vi "Raycaster_RunDDA.vi"(10 "Map Address":u32, 11 "DDA Calculation In":T1) -> (3 "DDA Calculation Out":T1)   [LabVIEW 2020]
uses:
  Controls/Raycaster_DDACalcs.ctl
  Controls/Raycaster_WallColumnAxis.ctl
  Globals/FGV_TileVisibleEnum.ctl
  Map_GetMaps.vi
  <vilib>/Utility/file.llb/Application Directory.vi
  <vilib>/rvi/DataTransferAndStorage/Container/XNode/niFpgaContainer.xnode
  <vilib>/rvi/Memory/Memory_Emulation/nirvimemoryFastEmulation.vi
  <vilib>/rvi/Memory/Memory_Emulation/nirvimemoryEmulation.vi
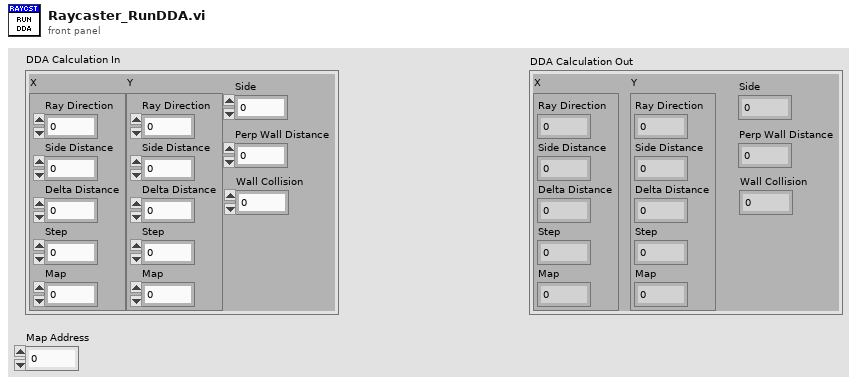
[diagram p1: front panel]
types:
  T1 = typedef "Raycaster_DDACalcs.ctl" = cluster{"X":T2, "Y":T2, "Side":u8, "Perp Wall Distance":fxp<+/-,32,16>, "Wall Collision":u8}
  T2 = typedef "Raycaster_WallColumnAxis.ctl" = cluster{"Ray Direction":fxp<+/-,32,16>, "Side Distance":fxp<+/-,32,16>, "Delta Distance":fxp<+/-,32,16>, "Step":i16, "Map":i16}
  T3 = typedef "FGV_TileVisibleEnum.ctl" = enum16{"Reset", "Set Value", "Read Value"}
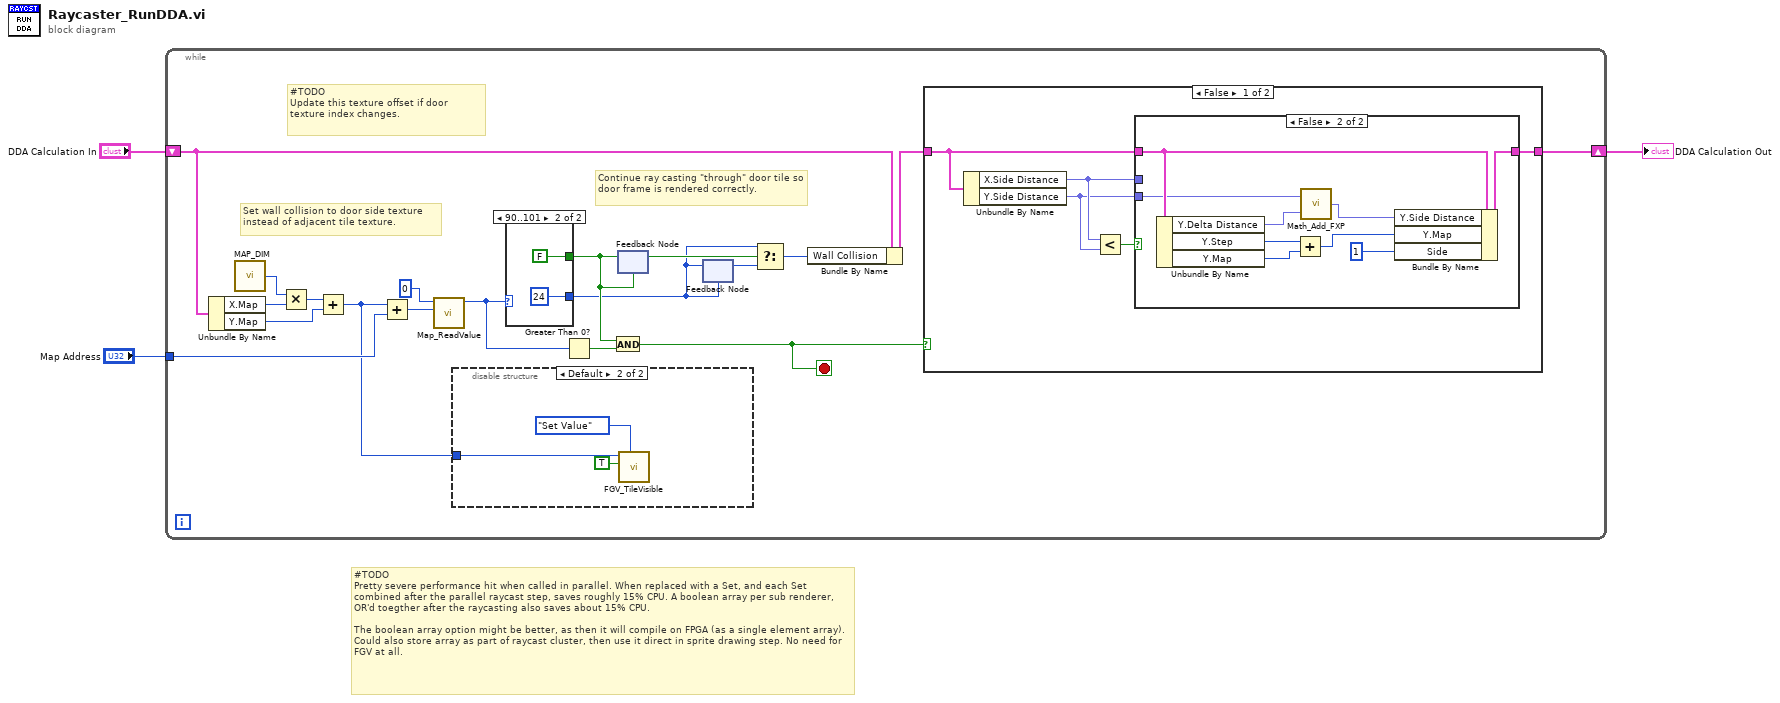
[diagram p0: block diagram]
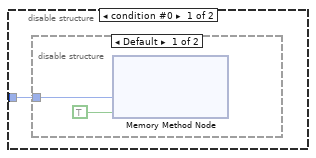
[diagram p2: hidden frame]
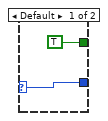
[diagram p4: hidden frame]
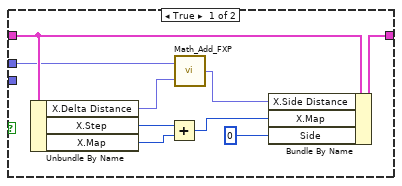
[diagram p5: hidden frame]
diagram:
  # "#TODO\nPretty severe performance hit when called in parallel. When replaced with a Set, and each Set combined after the parallel raycast step, saves roughly 15% CPU. A boolean array per sub renderer, OR'd toegther after the raycasting also saves about 15% CPU.\n\nThe boolean array option might be better, as then it will compile on FPGA (as a single element array). Could also store array as part of raycast cluster, then use it direct in sprite drawing step. No need for FGV at all."
  n1 = while {
    shift-right: [w15] -> w2
    shift-left: "DDA Calculation In" -> [w11]
    tunnel: "Map Address" -> [w6]
    stop <- w9 stop-if-true
    # "#TODO\nUpdate this texture offset if door texture index changes."
    # "Set wall collision to door side texture instead of adjacent tile texture."
    # "Continue ray casting \"through\" door tile so door frame is rendered correctly."
    n2 = Unbundle By Name(w11) -> ("X.Map"=w22:i16, "Y.Map"=w20:i16)
    n3 = call "MAP_DIM.vi"() -> ("MAP_DIM"=w19:i16)
    n4 = Multiply(x=w19, y=w22) -> (x*y=w21:i16)
    n5 = Add(x=w21, y=w20) -> (x+y=w4:i16)
    n6 = Add(x=w4, y=w6) -> (x+y=w5:u32)
    n7 = call "Map_ReadValue.vi"("Address"=w5, "Plane"=u8 0) -> ("Value"=w16:u8)  [unwired: 9 in]
    n8 = disable-structure shown="Default" {
      disable-tunnel: w4 -> [w23 w27]
      frame condition #0 {
        n9 = disable-structure shown="Default" {
          disable-tunnel: w23 -> [w25 _]
          frame condition #0 (active) {
            n10 = xnode ("Memory Method Node")("Address"=w25, "Data"=TRUE) -> ()  [unwired: 1 in, 1 out]
          }
          frame condition #1 {
          }
        }
      }
      frame condition #1 (active) {
        n11 = call "FGV_TileVisible.vi"("Tile Visible FGV"=FGV_TileVisibleEnum."Set Value", "Value"=TRUE, "Index"=w27) -> ()  [unwired: 8 in, 1 out]
      }
    }
    n12 = case shown="90..101" w16 {
      selector: w16 -> [w30 _]
      tunnel: [w30 u8 24 ("Value")] -> w7
      tunnel: [TRUE FALSE] -> w8
      frame Default {
      }
      frame 90..101 {
      }
    }
    n13 = Greater Than 0?(x=w16) -> (x > 0?=w17:bool)
    n14 = And(x=w8, y=w17) -> (x .and. y?=w9:bool)
    n15 = feedback #1(w8) -> (w13:bool)
    n16 = feedback-in #1(w8) -> ()
    n17 = feedback #2(w7) -> (w14:u8)
    n18 = feedback-in #2(w7) -> ()
    n19 = Select(t=w7, s=w13, f=w14) -> (s? t:f=w12:u8)
    n20 = Bundle By Name(cluster=w11, "Wall Collision"=w12) -> (w10:T1)
    n21 = case shown="False" w9 {
      tunnel: w10 -> [w34 w56]
      tunnel: [w33 w56] -> w15
      frame False {
        n22 = Unbundle By Name(w34) -> ("X.Side Distance"=w36:fxp<+/-,32,16>, "Y.Side Distance"=w35:fxp<+/-,32,16>)
        n23 = Less?(x=w36, y=w35) -> (x < y?=w37:bool)
        n24 = case shown="False" w37 {
          tunnel: w34 -> [w46 w55]
          tunnel: w36 -> [w40 _]
          tunnel: [w41 w50] -> w33
          tunnel: w35 -> [_ w49]
          frame True {
            n25 = Unbundle By Name(w46) -> ("X.Delta Distance"=w39:fxp<+/-,32,16>, "X.Step"=w45:i16, "X.Map"=w44:i16)
            n26 = Add(x=w45, y=w44) -> (x+y=w43:i16)
            n27 = call "Math_Add_FXP.vi"("y"=w39, "x"=w40) -> ("x*y"=w38:fxp<+/-,32,16>)
            n28 = Bundle By Name(cluster=w46, "X.Side Distance"=w38, "X.Map"=w43, "Side"=u8 0) -> (w41:T1)
          }
          frame False {
            n29 = Unbundle By Name(w55) -> ("Y.Delta Distance"=w48:fxp<+/-,32,16>, "Y.Step"=w54:i16, "Y.Map"=w53:i16)
            n30 = Add(x=w54, y=w53) -> (x+y=w52:i16)
            n31 = call "Math_Add_FXP.vi"("y"=w48, "x"=w49) -> ("x*y"=w47:fxp<+/-,32,16>)
            n32 = Bundle By Name(cluster=w55, "Y.Side Distance"=w47, "Y.Map"=w52, "Side"=u8 1) -> (w50:T1)
          }
        }
      }
      frame True {
      }
    }
  }
  "DDA Calculation Out" <- w2
